vi "Manage Bomb.vi"(7 "Packed refs":T1, 8 "error in (no error)":errorcluster, 11 "Board Game in":refnum<class "Board Game.lvclass">) -> (0 "error out":errorcluster, 3 "Board Game out":refnum<class "Board Game.lvclass">)   [LabVIEW 2021, in "Board Game.lvclass"]
uses:
  Board Game.lvclass
  Application/Packed Refs.ctl
  GameEl_class/private/Enum Direction.ctl
  Board Game.lvclass/Board Game.ctl
  GameEl_class/GameEl.lvclass/GameEl.ctl
  Snake_class/Snake.lvclass/Snake.ctl
  Shield/Shield.lvclass/Shield.ctl
  Imposible_Snake_v2/LVApp/Modules/Sound Manager/Typedefs/Sound Effects.ctl
  GameEl_class/Read position.vi
  Snake_class/Write Bomb Crash.vi
  Shield/Read Shield Count.vi
  Snake_class/Read Star.vi
  GameEl_class/Read Visible.vi
  Bomb/Bomb.lvclass
  C:/Users/poche/Programs/LabVIEW/imposible snake/GameEl_class/GameEl.lvclass
  Snake_class/Snake.lvclass
  Shield/Shield.lvclass
  GameEl_class/GameEl.lvclass
  Imposible_Snake_v2/LVApp/Modules/Sound Manager/Sound Manager.lvlib
  Application/Game.lvclass
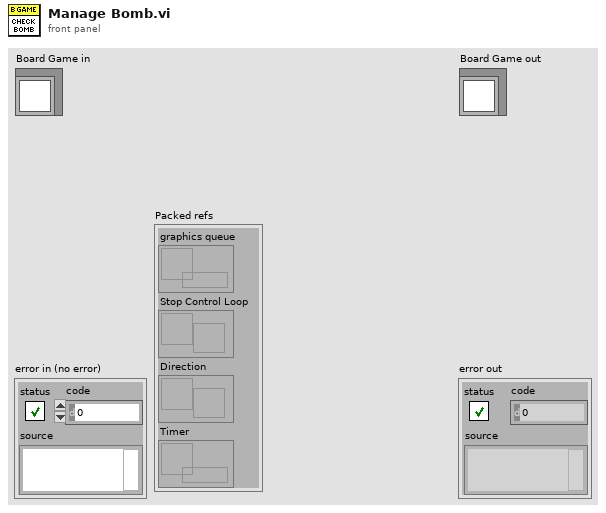
[diagram p1: front panel]
types:
  T1 = typedef "Game.lvclass/Packed Refs.ctl" = cluster{"graphics queue":refnum<queue>, "Stop Control Loop":refnum<user-event>, "Direction":refnum<notifier>, "Timer":refnum<data-value>}
  T2 = typedef "Sound Manager.lvlib/Sound Effects.ctl" = enum16{"Bomb In", "Bomb Out", "Bomb Touched", "Game Over", "Victory", "Eat", "10 Fruits", "Eat2", "Eat3", "Eat4", "MaxShield", "Shield", "10p", "Grape In", "Grape Out", "20p", "30p", "40p", "50p", "60p", "70p", "80p", "90p", "100p", "All shields cracked", "Mouse In", "Mouse Out", "Mouse Eaten", "Grape Eaten", "States Recover", "Broken Shield", "Bonus", "Happy Time", "explode", "Game over musica", "Back Music", "Shield Catch", "Evil lough", "Cricket In", "Cricket eaten", "Lets Go", "Jump1", "Jump2", "Jump3", "Unstoppable", "Troll Music", "winner", "menu"}
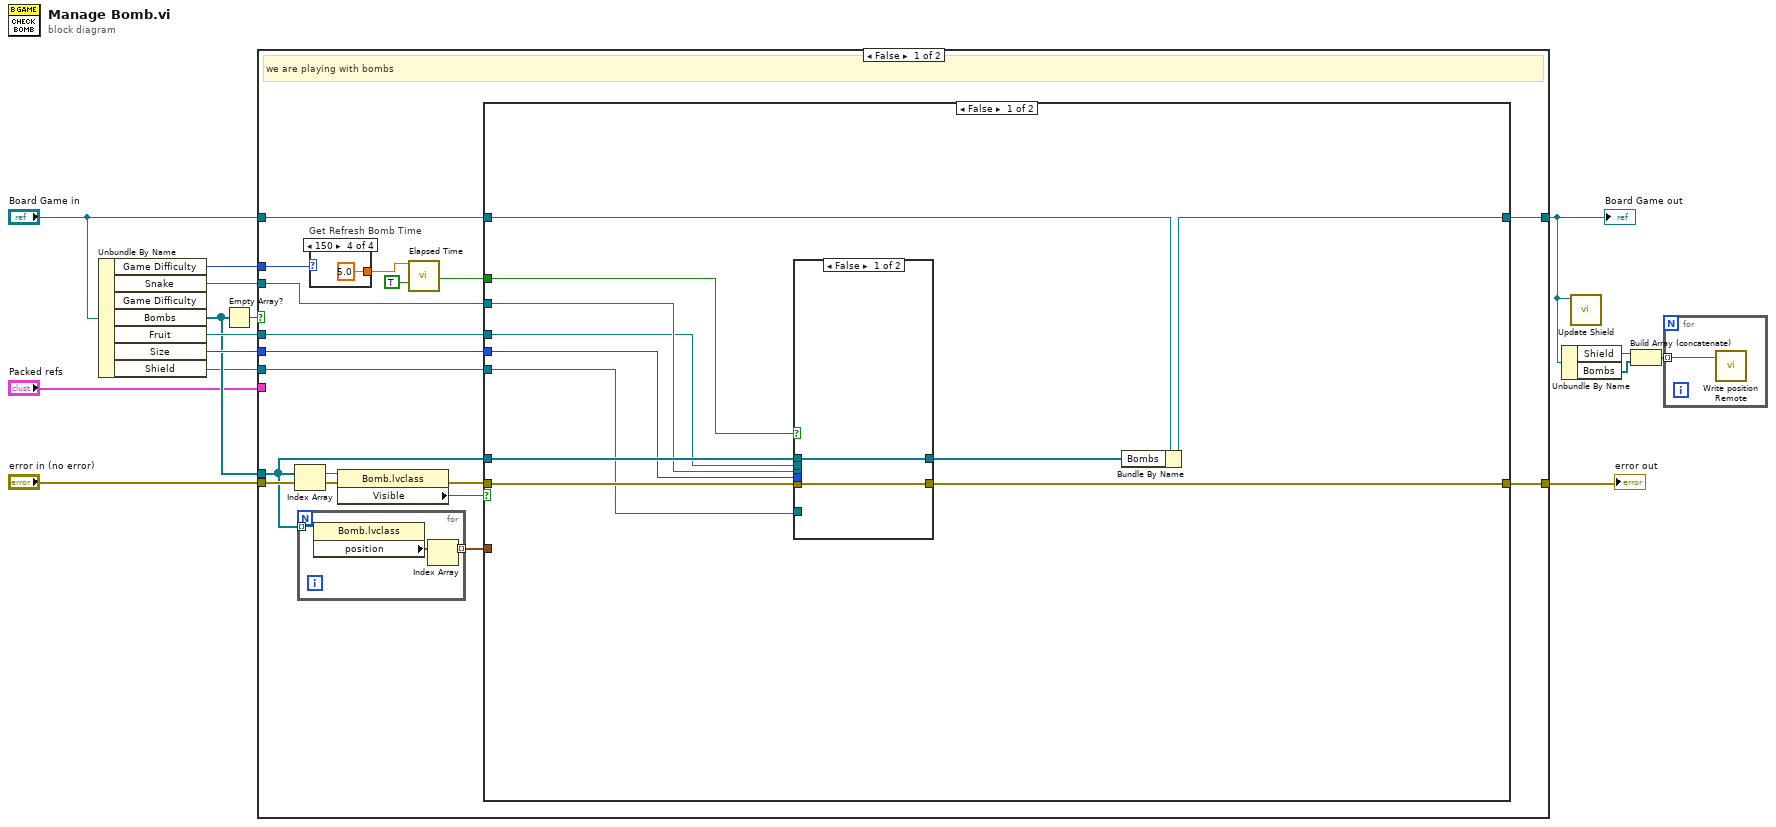
[diagram p0: block diagram]
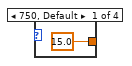
[diagram p2: hidden frame]
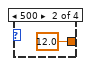
[diagram p3: hidden frame]
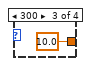
[diagram p4: hidden frame]
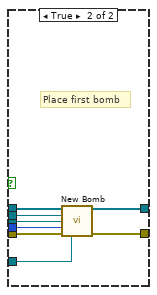
[diagram p5: hidden frame]
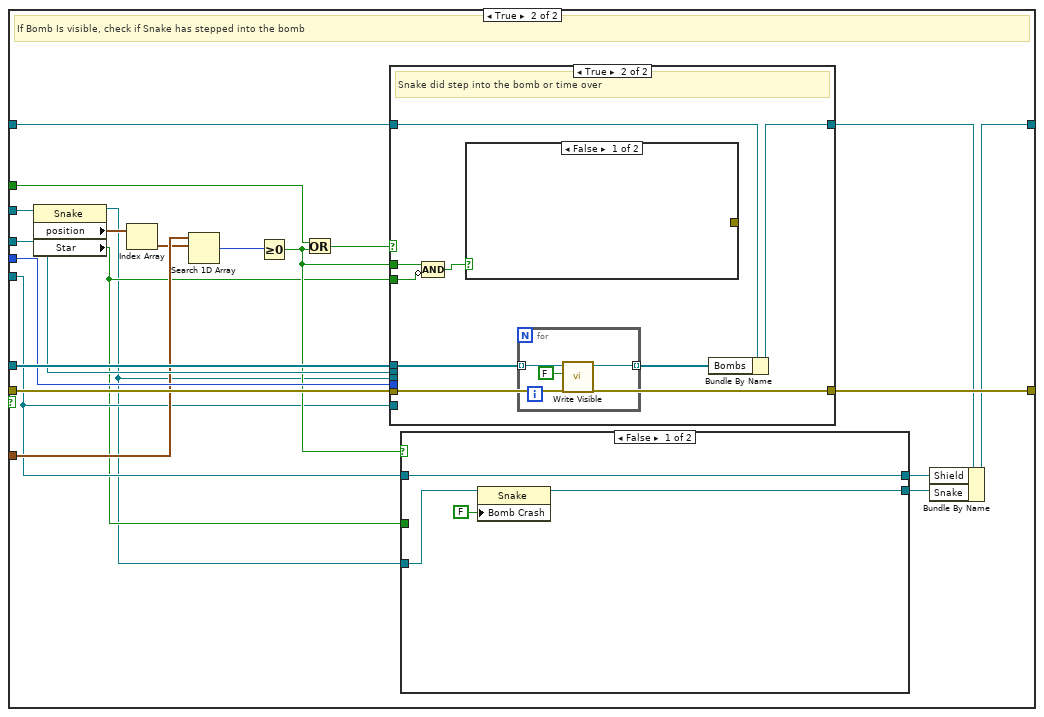
[diagram p6: hidden frame]
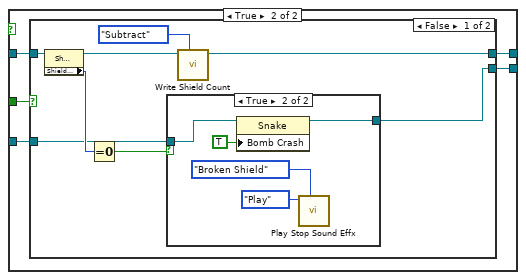
[diagram p7: hidden frame]
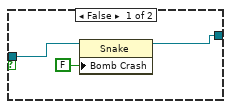
[diagram p8: hidden frame]
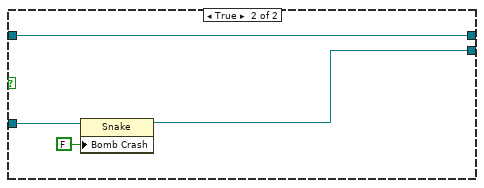
[diagram p9: hidden frame]
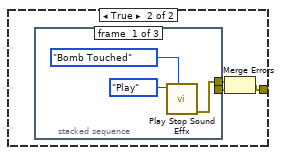
[diagram p11: hidden frame]
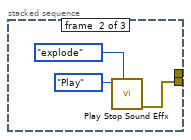
[diagram p12: hidden frame]
diagram:
  n1 = Unbundle By Name("Board Game in") -> ("Game Difficulty"=w13:u32, "Snake"=w12:refnum<class "Snake.lvclass">, "Bombs"=w8:refnum<class "Bomb.lvclass">[], "Fruit"=w10:refnum<class "Fruit.lvclass">, "Size"=w9:u16, "Shield"=w6:refnum<class "Shield.lvclass">)  [unwired: 1 out]
  n2 = Empty Array?(array=w8) -> (empty?=w7:bool)
  n3 = case shown="False" w7 {
    tunnel: [w32 w134] -> w5
    tunnel: "Board Game in" -> [w31 w134]
    tunnel: "error in (no error)" -> [w30 w133]
    tunnel: w13 -> [w27 _]
    tunnel: w12 -> [w25 _]
    tunnel: [w23 w133] -> w11
    tunnel: w10 -> [w21 _]
    tunnel: w9 -> [w20 _]
    tunnel: "Packed refs" -> [_ _]
    tunnel: w8 -> [w17 _]
    tunnel: w6 -> [w16 _]
    frame False {
      # "we are playing with bombs"
      n4 = Index Array(array=w17) -> (element=w19:refnum<class "Bomb.lvclass">)  [unwired: 1 in]
      n5 = for {
        tunnel: w17 -> [w35] mode=indexing
        tunnel: [w33] -> w18 mode=indexing
        n6 = property class="Bomb.lvclass"(reference=w35) -> ("position"=w34:cluster{"x":dbl, "y":dbl}[])  [unwired: 1 in, 2 out]
        n7 = Index Array(array=w34) -> (element=w33:cluster{"x":dbl, "y":dbl})  [unwired: 1 in]
      }
      n8 = case "Get Refresh Bomb Time" shown="150" w27 {
        tunnel: [15.0 ("double precision float") 12.0 ("double precision float") 10.0 ("double precision float") 5.0 ("double precision float")] -> w26
        frame 750, Default {
        }
        frame 500 {
        }
        frame 300 {
        }
        frame 150 {
        }
      }
      n9 = property class="Bomb.lvclass"(reference=w19, error in=w30) -> (error out=w29:errorcluster, "Visible"=w28:bool)  [unwired: 1 out]
      n10 = call "Elapsed Time"("Time Target (s)"=w26, "Auto Reset"=TRUE) -> ("Time has Elapsed"=w22:bool)  [unwired: 10 in, 7 out]
      n11 = case shown="False" w28 {
        tunnel: w31 -> [w50 w77]
        tunnel: [w42 w67] -> w32
        tunnel: w29 -> [w49 w79]
        tunnel: w25 -> [w46 w81]
        tunnel: w18 -> [_ w70]
        tunnel: [w48 w78] -> w23
        tunnel: w22 -> [w43 w74]
        tunnel: w17 -> [w47 w73]
        tunnel: w21 -> [w45 w72]
        tunnel: w20 -> [w44 w71]
        tunnel: w16 -> [w40 w64]
        frame False {
          n12 = case shown="False" w43 {
            tunnel: w49 -> [w52 w60]
            tunnel: [w52 w59] -> w48
            tunnel: w47 -> [w51 w58]
            tunnel: w46 -> [_ w57]
            tunnel: w45 -> [_ w56]
            tunnel: w44 -> [_ w55]
            tunnel: [w51 w54] -> w41
            tunnel: w40 -> [_ w53]
            frame False {
            }
            frame True {
              # "Place first bomb"
              n13 = call "New Bomb.vi"("Bomb in"=w58, "Fruit"=w56, "Snake"=w57, "B Game Size"=w55, "error in (no error)"=w60, "Shield"=w53) -> ("Bomb out"=w54:refnum<class "Bomb.lvclass">[], "error out"=w59:errorcluster)  [unwired: 7 in, 1 out]
            }
          }
          n14 = Bundle By Name(cluster=w50, "Bombs"=w41) -> (w42:refnum<class "Board Game.lvclass">)
        }
        frame True {
          # "If Bomb Is visible, check if Snake has stepped into the bomb"
          n15 = property class="Snake"(reference=w81) -> (reference out=w61:refnum<class "Snake.lvclass">, "position"=w80:cluster{"x":dbl, "y":dbl}[], "Star"=w62:bool)  [unwired: 1 in, 1 out]
          n16 = Index Array(array=w80) -> (element=w69:cluster{"x":dbl, "y":dbl})  [unwired: 1 in]
          n17 = Search 1D Array(1D array=w70, element=w69) -> (index of element=w68:i32)  [unwired: 1 in]
          n18 = Greater Or Equal To 0?(x=w68) -> (x >= 0?=w66:bool)
          n19 = Or(x=w74, y=w66) -> (x .or. y?=w75:bool)
          n20 = case shown="True" w75 {
            tunnel: w79 -> [w111 w116]
            tunnel: [w111 w116] -> w78
            tunnel: w77 -> [w112 w120]
            tunnel: [w112 w119] -> w76
            tunnel: w73 -> [_ w117]
            tunnel: w72 -> [_ _]
            tunnel: w61 -> [_ _]
            tunnel: w71 -> [_ _]
            tunnel: w66 -> [_ w118]
            tunnel: w64 -> [_ _]
            tunnel: w62 -> [_ w114]
            frame False {
              # "Snake avoided bomb and still not time to replace it"
            }
            frame True {
              # "Snake did step into the bomb or time over"
              n21 = Compound Arithmetic op=AND(w118, invert w114) -> (w115:bool)
              n22 = case shown="False" w115 {
                tunnel: [_ w125] -> _
                frame False {
                }
                frame True {
                  n23 = stacked-sequence {
                    tunnel: [_ w130 _] -> w126
                    tunnel: [w127 _ _] -> w124
                    frame #0 {
                      n24 = call "Play Stop Sound Effx.vi"("Sound Effect"=Sound_Effects."Bomb Touched", "Function"=enum16{"Play", "Stop"}."Play") -> ("error in (no error)"=w127:errorcluster)  [unwired: 9 in]
                    }
                    frame #1 {
                      n25 = call "Play Stop Sound Effx.vi"("Sound Effect"=Sound_Effects."explode", "Function"=enum16{"Play", "Stop"}."Play") -> ("error in (no error)"=w130:errorcluster)  [unwired: 9 in]
                    }
                    frame #2 {
                      # "play, broken\nshield"
                    }
                  }
                  n26 = Merge Errors(w124, w126) -> (w125:errorcluster)
                }
              }
              n27 = for {
                tunnel: w117 -> [w123] mode=indexing
                tunnel: [w122] -> w113 mode=indexing
                n28 = call "Write Visible.vi"("Visible"=FALSE, "GameEl in"=w123) -> ("GameEl out"=w122:refnum<class "Bomb.lvclass">)  [unwired: 8 in, 1 out]
              }
              n29 = Bundle By Name(cluster=w120, "Bombs"=w113) -> (w119:refnum<class "Board Game.lvclass">)
            }
          }
          n30 = case shown="False" w66 {
            tunnel: w64 -> [w85 w90]
            tunnel: [w85 w89] -> w65
            tunnel: [w82 w88] -> w63
            tunnel: w62 -> [_ w87]
            tunnel: w61 -> [w84 w86]
            frame False {
              n31 = property class="Snake"(reference=w84, "Bomb Crash"=FALSE) -> (reference out=w82:refnum<class "Snake.lvclass">)  [unwired: 1 in, 1 out]
            }
            frame True {
              n32 = case shown="False" w87 {
                tunnel: w90 -> [w98 w110]
                tunnel: [w94 w110] -> w89
                tunnel: [w91 w107] -> w88
                tunnel: w86 -> [w92 w108]
                frame False {
                  n33 = property class="Shield.lvclass"(reference=w98) -> (reference out=w97:refnum<class "Shield.lvclass">, "Shield Count"=w95:u8)  [unwired: 1 in, 1 out]
                  n34 = Equal To 0?(x=w95) -> (x = 0?=w93:bool)
                  n35 = case shown="True" w93 {
                    tunnel: w92 -> [w101 w106]
                    tunnel: [w99 w104] -> w91
                    frame False {
                      n36 = property class="Snake"(reference=w101, "Bomb Crash"=FALSE) -> (reference out=w99:refnum<class "Snake.lvclass">)  [unwired: 1 in, 1 out]
                    }
                    frame True {
                      n37 = property class="Snake"(reference=w106, "Bomb Crash"=TRUE) -> (reference out=w104:refnum<class "Snake.lvclass">)  [unwired: 1 in, 1 out]
                      n38 = call "Play Stop Sound Effx.vi"("Sound Effect"=Sound_Effects."Broken Shield", "Function"=enum16{"Play", "Stop"}."Play") -> ()  [unwired: 9 in, 1 out]
                    }
                  }
                  n39 = call "Write Shield Count.vi"("function"=enum16{"Add", "Subtract"}."Subtract", "Shield in"=w97) -> ("Shield out"=w94:refnum<class "Shield.lvclass">)  [unwired: 8 in, 1 out]
                }
                frame True {
                  n40 = property class="Snake"(reference=w108, "Bomb Crash"=FALSE) -> (reference out=w107:refnum<class "Snake.lvclass">)  [unwired: 1 in, 1 out]
                }
              }
            }
          }
          n41 = Bundle By Name(cluster=w76, "Shield"=w65, "Snake"=w63) -> (w67:refnum<class "Board Game.lvclass">)
        }
      }
    }
    frame True {
      # "we are not playing with bombs"
    }
  }
  "error out" <- w11
  "Board Game out" <- w5
  n42 = Unbundle By Name(w5) -> ("Shield"=w4:refnum<class "Shield.lvclass">, "Bombs"=w3:refnum<class "Bomb.lvclass">[])
  n43 = call "Update Shield.vi"("Board Game in"=w5) -> ()  [unwired: 11 in]
  n44 = Build Array (concatenate)(w4, w3) -> (w2:refnum<class "GameEl.lvclass">[])
  n45 = for {
    tunnel: w2 -> [w135] mode=indexing
    n46 = call "Write position Remote.vi"("GameEl in"=w135) -> ()  [unwired: 10 in, 1 out]
  }
